vi "Program_Load.vi"(8 "error in (no error)":errorcluster, 9 "Time Start":dbl[unit], 10 "Array":dbl[][](array[numeric]), 11 "SpinCoater in":refnum<class "SpinCoater.lvclass">) -> (0 "error out":errorcluster, 3 "SpinCoater out":refnum<class "SpinCoater.lvclass">)   [LabVIEW 2018, in "SpinCoater.lvclass"]
uses:
  <instrlib>/Classes/SpinCoater/SpinCoater.lvclass
panel:
  out "read buffer":string
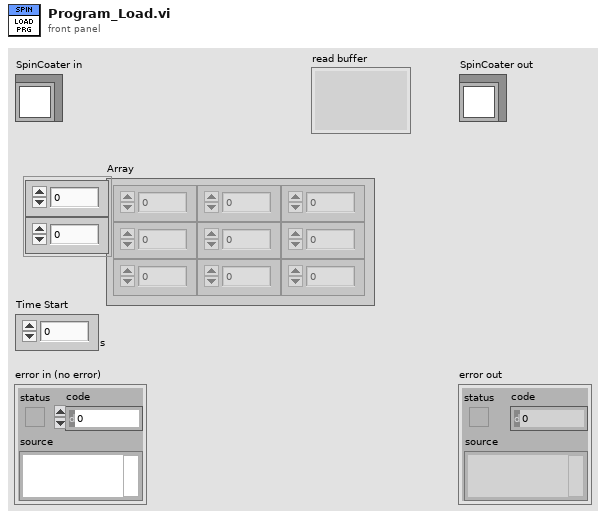
[diagram p1: front panel]
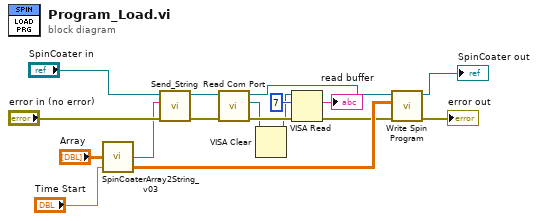
[diagram p0: block diagram]
diagram:
  n1 = call <instrlib>:"SpinCoaterArray2String_v03.vi"("Time Start"="Time Start", "Program Spin Coater\nSpeed (rpm)          Time (s)"="Array") -> ("Prg Spin Coater small"=w12:dbl[][], "remote control String"=w13:string)  [unwired: 2 in]
  n2 = call-dynamic "Send_String.vi"("error in (no error)"="error in (no error)", "String"=w13, "SpinCoater in"="SpinCoater in") -> ("error out"=w9:errorcluster, "SpinCoater out"=w8:refnum<class "SpinCoater.lvclass">)  [unwired: 7 in]
  n3 = call-dynamic "Read Com Port.vi"("error in (no error)"=w9, "SpinCoater in"=w8) -> ("error out"=w7:errorcluster, "Com Port"=w2:refnum<visa-resource-name>, "SpinCoater out"=w6:refnum<class "SpinCoater.lvclass">)  [unwired: 7 in]
  n4 = VISA Clear(VISA resource name=w2) -> (VISA resource name out=w1:refnum<visa-resource-name>)  [unwired: 1 in, 1 out]
  n5 = VISA Read(VISA resource name=w1, byte count=u32 7, error in (no error)=w7) -> (read buffer=→"read buffer":string, error out=w5:errorcluster)  [unwired: 2 out]
  n6 = call-dynamic "Write Spin Program.vi"("error in (no error)"=w5, "Spin Program"=w12, "SpinCoater in"=w6) -> ("error out"=→"error out":errorcluster, "SpinCoater out"=→"SpinCoater out":refnum<class "SpinCoater.lvclass">)  [unwired: 7 in]
